vi "new.vi"(8 "error in (no error)":errorcluster, 10 "messageIn":refnum<user-event>, 11 "description":string) -> (0 "error out":errorcluster, 3 "ExampleTask_MsgUserEventStopNotifier Out":refnum<class "ExampleTask_MsgUserEventStop.lvclass">)   [LabVIEW 2023, in "ExampleTask_MsgUserEventStop.lvclass"]
doc: "Constructor"
uses:
  ExampleTask_MsgUserEventStop.lvclass
  ExampleTask_MsgUserEventStop.lvclass/ExampleTask_MsgUserEventStop.ctl
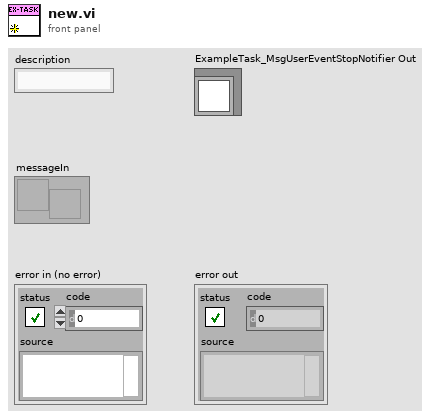
[diagram p1: front panel]
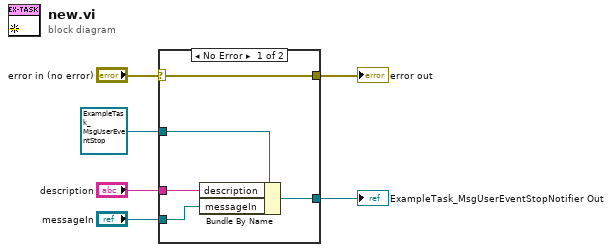
[diagram p0: block diagram]
diagram:
  n1 = case shown="No Error" "error in (no error)" {
    selector: "error in (no error)" -> [w11 w13]
    tunnel: [w11 w13] -> w5
    tunnel: [w10 w12] -> w3
    tunnel: refnum<class "ExampleTask_MsgUserEventStop.lvclass"> refnum ("ExampleTask_StopNotifier in") -> [w9 w12]
    tunnel: "description" -> [w8 _]
    tunnel: "messageIn" -> [w7 _]
    frame No Error {
      n2 = Bundle By Name(cluster=w9, "description"=w8, "messageIn"=w7) -> (w10:refnum<class "ExampleTask_MsgUserEventStop.lvclass">)
    }
    frame Error {
    }
  }
  "error out" <- w5
  "ExampleTask_MsgUserEventStopNotifier Out" <- w3
